vi "PicoScope2000aRunBlock.vi"(7 "Acquisition Settings":T1={"preTriggerSamples"=0, "postTriggerSamples"=1000, "timebase"=2} {"postTriggerSamples" format="%_6p"; "preTriggerSamples" format="%_6p"}, 8 "error in (no error)":errorcluster, 11 "handle in":i16) -> (0 "error out":errorcluster, 3 "handle out":i16, 4 "timeIndisposedMs":dbl, 6 "Total Requested Samples":u64)   [LabVIEW 2010]
doc: "Calls RunBlock"
uses:
  ps2000a.dll
  shared/Acquisition Settings.ctl
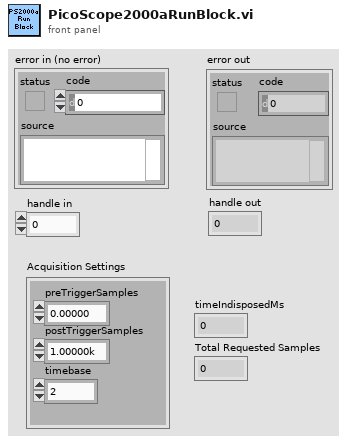
[diagram p1: front panel]
types:
  T1 = typedef "Acquisition Settings.ctl" = cluster{"preTriggerSamples":u64, "postTriggerSamples":u64, "timebase":u32}
  T2 = cluster{"status":bool, "code":u32, "source":string}
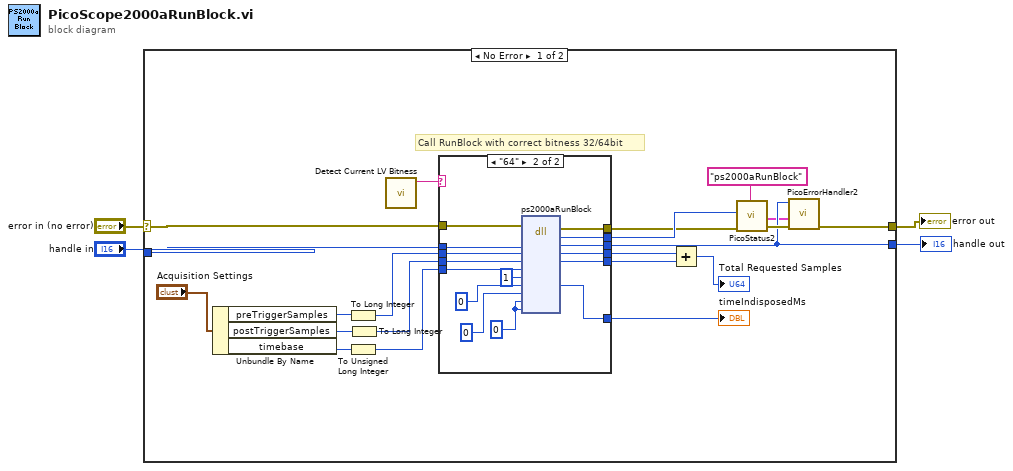
[diagram p0: block diagram]
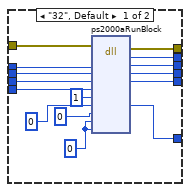
[diagram p2: hidden frame]
diagram:
  n1 = case shown="No Error" "error in (no error)" {
    selector: "error in (no error)" -> [w19 w57]
    tunnel: [w15 w57] -> w2
    tunnel: "handle in" -> [w18 w56]
    tunnel: [w14 w56] -> w3
    frame No Error {
      # "Call RunBlock with correct bitness 32/64bit"
      n2 = Unbundle By Name("Acquisition Settings") -> ("preTriggerSamples"=w11:u64, "postTriggerSamples"=w9:u64, "timebase"=w10:u32)
      n3 = To Long Integer(number=w11) -> (32bit integer=w8:i32)
      n4 = To Unsigned Long Integer(number=w10) -> (unsigned 32bit integer=w6:u32)
      n5 = To Long Integer(number=w9) -> (32bit integer=w7:i32)
      n6 = call "Detect Current LV Bitness.vi"() -> ("bitness"=w16:string)  [unwired: 11 in]
      n7 = case shown="\"64\"" w16 {
        tunnel: [w40 w55] -> w25
        tunnel: [w39 w54] -> w24
        tunnel: [w38 w53] -> w22
        tunnel: [w37 w52] -> w21
        tunnel: w19 -> [w36 w51]
        tunnel: w18 -> [w35 w50]
        tunnel: w8 -> [w33 w48]
        tunnel: w7 -> [w32 w47]
        tunnel: w6 -> [w31 w46]
        tunnel: [w30 w45] -> w14
        tunnel: [w27 w43] -> w13
        frame "32", Default {
          w29 = u32 0 ("pParameter")
          n8 = dll-call lib="ps2000a.dll" fn="ps2000aRunBlock" ("ps3000.dll:_ps3000_open_unit@0")(error in=w36, "handle"=w35, "noOfPreTriggerSamples"=w33, "noOfPostTriggerSamples"=w32, "timebase"=w31, "oversample"=i16 1, "timeIndisposedMs"=0 ("pParameter"), "segmentIndex"=u32 0, "lpReady"=w29, "pParameter"=w29) -> (error out=w37:errorcluster, "PICO_STATUS"=w38:u32, "handle"=w30:i16, "noOfPreTriggerSamples"=w40:i32, "noOfPostTriggerSamples"=w39:i32, "timeIndisposedMs"=w27:i32)  [unwired: 7 in, 1 out]
        }
        frame "64" {
          w44 = u64 0 ("pParameter")
          n9 = dll-call lib="ps2000a.dll" fn="ps2000aRunBlock" ("ps3000.dll:_ps3000_open_unit@0")(error in=w51, "handle"=w50, "noOfPreTriggerSamples"=w48, "noOfPostTriggerSamples"=w47, "timebase"=w46, "oversample"=i16 1, "timeIndisposedMs"=0 ("pParameter"), "segmentIndex"=u32 0, "lpReady"=w44, "pParameter"=w44) -> (error out=w52:errorcluster, "PICO_STATUS"=w53:u32, "handle"=w45:i16, "noOfPreTriggerSamples"=w55:i32, "noOfPostTriggerSamples"=w54:i32, "timeIndisposedMs"=w43:i32)  [unwired: 7 in, 1 out]
        }
      }
      "timeIndisposedMs" <- w13
      n10 = Add(x=w25, y=w24) -> (x+y=→"Total Requested Samples":i32)
      n11 = call "PicoStatus2.vi"("PICO source"="ps2000aRunBlock" ("source"), "Error in"=w21, "PICO STATUS"=w22) -> ("error out"=w17:errorcluster, "PICO_STATUS out"=w5:T2)  [unwired: 5 in]
      n12 = call "PicoErrorHandler2.vi"("error in (no error)"=w17, "PICO_STATUS in"=w5, "handle In"=w14) -> ("error out"=w15:errorcluster)  [unwired: 8 in]
    }
    frame Error {
    }
  }
  "error out" <- w2
  "handle out" <- w3
